vi "GlobalGetHeidenhainDriftOnOff.vi"() -> ()   [LabVIEW 2013]
panel:
  out "GetDrift":bool
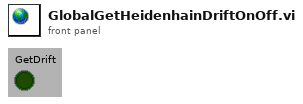
[diagram p1: front panel]
diagram:
